vi "Create Generic Dev Obj.vi"(8 "error in (no error)":errorcluster, 11 "DevInfo in":refnum<class "DevInfo.lvclass">) -> (0 "error out":errorcluster, 2 "Generic Dev Obj":refnum<class "Hardware.lvclass">, 3 "DevInfo out":refnum<class "DevInfo.lvclass">)   [LabVIEW 2016, in "Hardware.lvlib" / "DevInfo.lvclass"]
uses:
  <userlib>/Common Components/Hardware/DevInfo/DevInfo.lvclass
  <userlib>/Common Components/Hardware/Hardware.lvclass
  <userlib>/Common Components/Hardware/Hardware.lvclass/Hardware.ctl
  <userlib>/Common Components/Hardware/Write DevInfo.vi
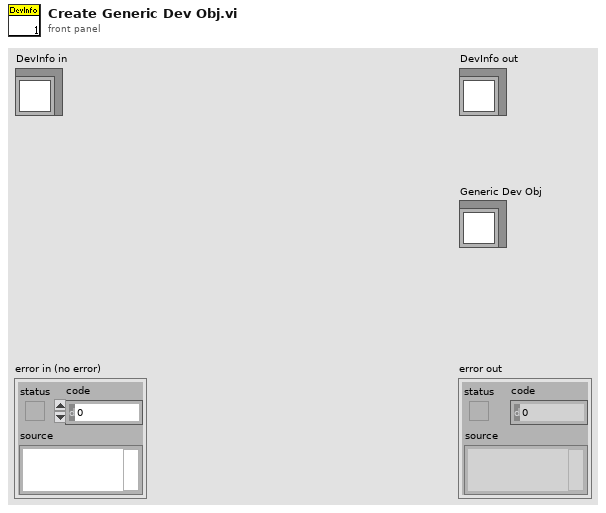
[diagram p1: front panel]
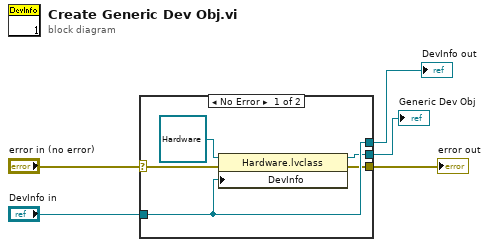
[diagram p0: block diagram]
diagram:
  n1 = case shown="No Error" "error in (no error)" {
    selector: "error in (no error)" -> [w9 w12]
    tunnel: [w6 w12] -> w4
    tunnel: [w8 w11] -> w2
    tunnel: "DevInfo in" -> [w8 w11]
    tunnel: [w7 _] -> w1
    frame No Error {
      n2 = property class="Hardware.lvclass"(reference=refnum<class "Hardware.lvclass"> refnum ("Hardware.lvlib:Hardware.lvclass"), error in=w9, "DevInfo"=w8) -> (reference out=w7:refnum<class "Hardware.lvclass">, error out=w6:errorcluster)
    }
    frame Error {
    }
  }
  "error out" <- w4
  "DevInfo out" <- w2
  "Generic Dev Obj" <- w1
